vi "Read Zstate T.vi"(11 "HE1_Z_state in":refnum<class "HE_Z_state_v2.lvclass">) -> (2 "T (ms)":u32, 3 "HE1_Z_state out":refnum<class "HE_Z_state_v2.lvclass">)   [LabVIEW 2019, in "Heating.lvlib" / "HE_Z_state_v2.lvclass"]
uses:
  HE_Z_state_v2.lvclass
  HE_Z_state_v2.lvclass/HE_Z_state_v2.ctl
  Sequence/State/State.lvclass/State.ctl
  Sequence/State/State.lvclass
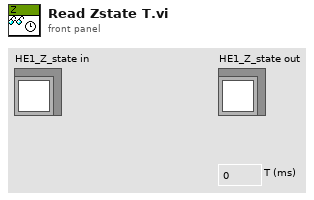
[diagram p1: front panel]
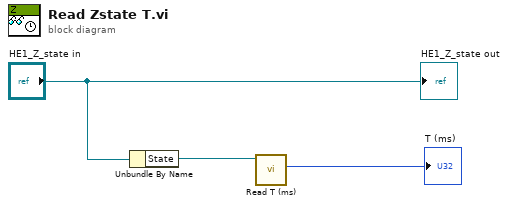
[diagram p0: block diagram]
diagram:
  n1 = Unbundle By Name("HE1_Z_state in") -> ("State"=w1:refnum<class "State.lvclass">)
  n2 = call "Read T (ms).vi"("State in"=w1) -> ("T (ms)"=→"T (ms)":u32)  [unwired: 9 in, 1 out]
  "HE1_Z_state out" <- "HE1_Z_state in"
